vi "SH_calcDistance2.vi"(1 "Shapelet 2":dbl[](array[numeric]), 3 "Shapelet 1":dbl[](array[numeric])) -> (0 "Distance out":dbl)   [LabVIEW 2016, in "Shapelets Search (Brute Force).lvlib"]
uses:
  Shapelets Search (Brute Force).lvlib
panel:
  # "This VI is a part of BCI Design library, http://www.ru-bci.org \nCopyright © 2020, Sotnikov Peter, All rights reserved. License: CC BY-NC 4.0"
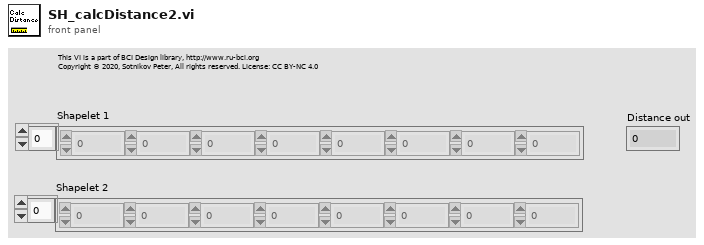
[diagram p1: front panel]
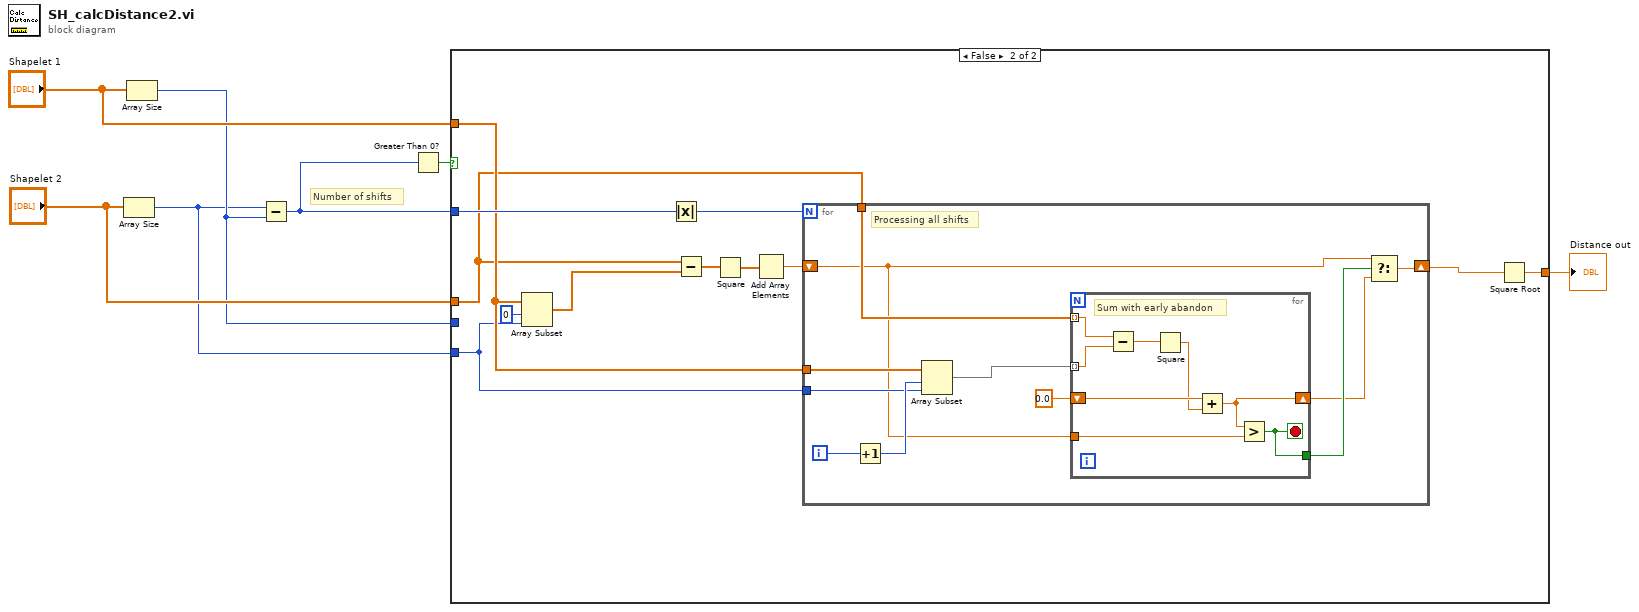
[diagram p0: block diagram]
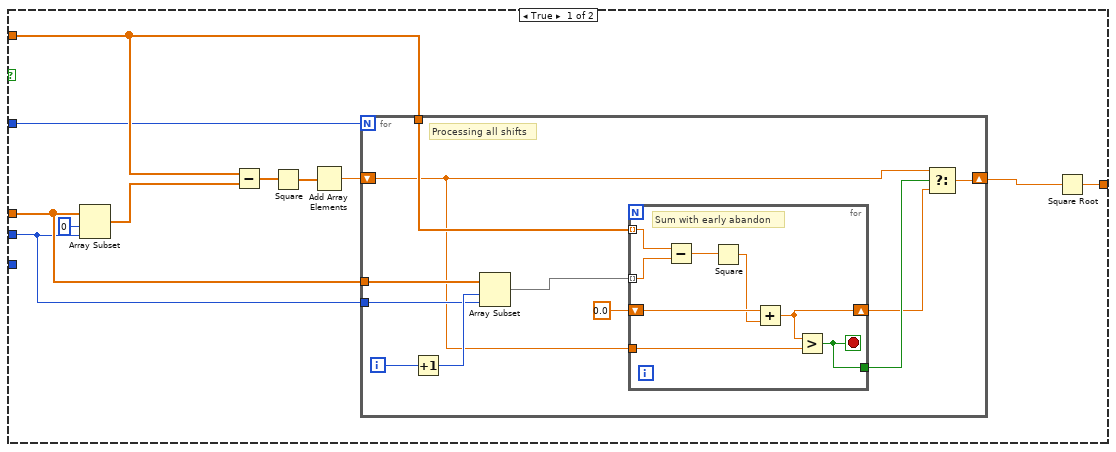
[diagram p2: hidden frame]
diagram:
  # "Number of shifts"
  n1 = Array Size(array="Shapelet 2") -> (size(s)=w1:i32)
  n2 = Array Size(array="Shapelet 1") -> (size(s)=w5:i32)
  n3 = Subtract(x=w1, y=w5) -> (x-y=w3:i32)
  n4 = Greater Than 0?(x=w3) -> (x > 0?=w2:bool)
  n5 = case shown="False" w2 {
    tunnel: "Shapelet 1" -> [w14 w41]
    tunnel: "Shapelet 2" -> [w13 w40]
    tunnel: w5 -> [w12 _]
    tunnel: [w11 w45] -> w4
    tunnel: w3 -> [w9 w43]
    tunnel: w1 -> [_ w39]
    frame True {
      n6 = Array Subset(array=w13, index=0, length=w12) -> (w10:dbl[])
      n7 = Subtract(x=w14, y=w10) -> (x-y=w17:dbl[])
      n8 = Square(x=w17) -> (x^2=w16:dbl[])
      n9 = Add Array Elements(numeric array=w16) -> (sum=w15:dbl)
      n10 = for {
        N: w9 -> [_]
        shift-right: [w23] -> w8
        shift-left: w15 -> [w22]
        tunnel: w14 -> [w25]
        tunnel: w13 -> [w29]
        tunnel: w12 -> [w26]
        i -> [w28]
        # "Processing all shifts"
        n11 = Increment(x=w28) -> (x+1=w27:i32)
        n12 = Array Subset(array=w29, index=w27, length=w26) -> (w19:dbl[])
        n13 = for {
          tunnel: w25 -> [w36] mode=indexing
          tunnel: w19 -> [w35] mode=indexing
          shift-right: [w32] -> w20
          shift-left: 0.0 -> [w34]
          tunnel: w22 -> [w31]
          tunnel: [w30] -> w21
          stop <- w30 stop-if-true
          # "Sum with early abandon"
          n14 = Subtract(x=w36, y=w35) -> (x-y=w37:dbl)
          n15 = Square(x=w37) -> (x^2=w33:dbl)
          n16 = Add(x=w34, y=w33) -> (x+y=w32:dbl)
          n17 = Greater?(x=w32, y=w31) -> (0:w30:bool)
        }
        n18 = Select(t=w22, s=w21, f=w20) -> (s? t:f=w23:dbl)
      }
      n19 = Square Root(x=w8) -> (sqrt(x)=w11:dbl)
    }
    frame False {
      n20 = Array Subset(array=w41, index=0, length=w39) -> (w44:dbl[])
      n21 = Absolute Value(x=w43) -> (abs(x)=w42:i32)
      n22 = Subtract(x=w40, y=w44) -> (x-y=w48:dbl[])
      n23 = Square(x=w48) -> (x^2=w47:dbl[])
      n24 = Add Array Elements(numeric array=w47) -> (sum=w46:dbl)
      n25 = for {
        N: w42 -> [_]
        shift-right: [w54] -> w38
        shift-left: w46 -> [w53]
        tunnel: w40 -> [w56]
        tunnel: w41 -> [w60]
        tunnel: w39 -> [w57]
        i -> [w59]
        # "Processing all shifts"
        n26 = Increment(x=w59) -> (x+1=w58:i32)
        n27 = Array Subset(array=w60, index=w58, length=w57) -> (w50:dbl[])
        n28 = for {
          tunnel: w56 -> [w67] mode=indexing
          tunnel: w50 -> [w66] mode=indexing
          shift-right: [w63] -> w51
          shift-left: 0.0 -> [w65]
          tunnel: w53 -> [w62]
          tunnel: [w61] -> w52
          stop <- w61 stop-if-true
          # "Sum with early abandon"
          n29 = Subtract(x=w67, y=w66) -> (x-y=w68:dbl)
          n30 = Square(x=w68) -> (x^2=w64:dbl)
          n31 = Add(x=w65, y=w64) -> (x+y=w63:dbl)
          n32 = Greater?(x=w63, y=w62) -> (0:w61:bool)
        }
        n33 = Select(t=w53, s=w52, f=w51) -> (s? t:f=w54:dbl)
      }
      n34 = Square Root(x=w38) -> (sqrt(x)=w45:dbl)
    }
  }
  "Distance out" <- w4
